vi "setSamplingFsMode.vi"(8 "error in (no error)":errorcluster, 10 "Fs Mode":T1, 11 "Instrument.Lockin in":refnum<class "Instrument.Lockin.lvclass">) -> (0 "error out":errorcluster, 3 "Instrument.Lockin out":refnum<class "Instrument.Lockin.lvclass">)   [LabVIEW 2019, in "Instrument.Lockin.lvclass"]
doc: "Set the Sampling Fs Mode {Manual, Auto Fs, Max Fs}\n\nIf address=\"\", this API reads from localhost\nIf address is remote lockin, you need to add this computer to allowed whitelist on the lockin computer you are trying to access."
uses:
  Instrument.Lockin.lvclass
  <userlib>/LevyLab/Instrument Framework/Instrument Types/Lockin/Typedefs/LockinAPI.Sampling.FsMode--enum.ctl
  Typedefs/API/Lockin.setSamplingFsMode--cluster.ctl
  Instrument.DAQ/Typedefs/DAQ.Sampling.Fs Mode--enum.ctl
  Typedefs/API/Lockin.Commands--Enum.ctl
  Instrument.DAQ/Instrument.DAQ.lvclass
  <userlib>/LevyLab/Instrument Framework/Instrument Types/Lockin/Instrument.LockinAPI.lvclass
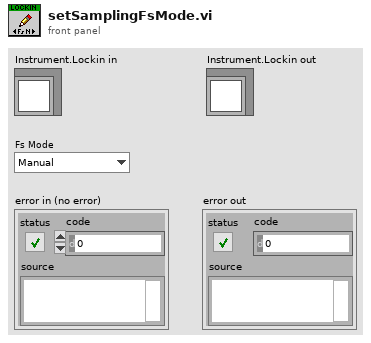
[diagram p1: front panel]
types:
  T1 = typedef "Instrument.LockinAPI.lvclass/LockinAPI.Sampling.FsMode--enum.ctl" = enum16{"Manual", "Auto Fs", "Max Fs"}
  T2 = typedef "Instrument.Lockin.lvclass/Lockin.Commands--Enum.ctl" = enum16{"setAO", "setAO_Amplitude", "setAO_DC", "setAO_Frequency", "setAO_Phase", "setAO_Function", "setREF", "setREF_Frequency", "setREF_Phase", "setREF_TC", "setREF_Roll-Off", "setDAQ", "setSampling", "setState", "getState", "getAO", "getAI", "getResults", "getSampling", "getAOconfig", "getREFconfig", "setInputGain", "setOutputGain", "getInputGain", "getOutputGain", "setSamplingFsMode", "getSamplingFsMode", "setSweep", "setSweep_Time", "setSweep_Table", "getStatus", "getSweepResults", "getSweepWaveforms", "startSweep", "stopSweep"}
  T3 = typedef "Instrument.Lockin.lvclass/Lockin.setSamplingFsMode--cluster.ctl" = cluster{"FsMode":T4}
  T4 = typedef "Instrument.DAQ.lvclass/DAQ.Sampling.Fs Mode--enum.ctl" = enum16{"Manual", "Auto Fs", "Max Fs"}
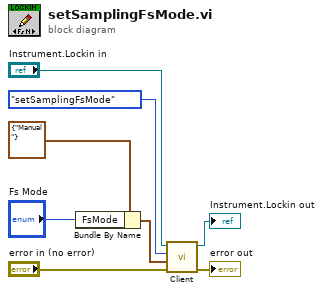
[diagram p0: block diagram]
diagram:
  n1 = Bundle By Name(cluster=T3 {"FsMode"=enum."Manual"} ("setSampleFsMode"), "FsMode"="Fs Mode") -> (w2:T3)
  n2 = call-dynamic "Client.vi"("error in (no error)"="error in (no error)", "Data in"=w2, "Command in"=Lockin.Commands--Enum."setSamplingFsMode" ("Commands"), "Instrument in"="Instrument.Lockin in") -> ("error out"=→"error out":errorcluster, "Instrument out"=→"Instrument.Lockin out":refnum<class "Instrument.Lockin.lvclass">)  [unwired: 4 in, 2 out]
